vi "Create from Info.vi"(8 "error in (no error)":errorcluster, 9 "Folder":path, 10 "Package Info":T1, 11 "NamedPackage in":refnum<class "NamedPackage.lvclass">) -> (0 "error out":errorcluster, 3 "NamedPackage out":refnum<class "NamedPackage.lvclass">)   [LabVIEW 2020, in "GPack.lvlib" / "NamedPackage.lvclass"]
uses:
  NamedPackage.lvclass
  Package Info.ctl
  NamedPackage.lvclass/NamedPackage.ctl
  GPack.lvlib
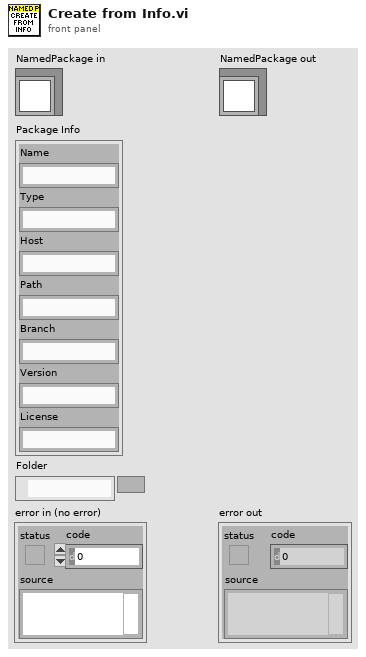
[diagram p1: front panel]
types:
  T1 = typedef "GPack.lvlib/Package Info.ctl" = cluster{"Name":string, "Type":string, "Host":string, "Path":string, "Branch":string, "Version":string, "License":string}
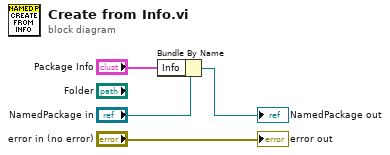
[diagram p0: block diagram]
diagram:
  n1 = Bundle By Name(cluster="NamedPackage in", "Info"="Package Info") -> (→"NamedPackage out":refnum<class "NamedPackage.lvclass">)
  "error out" <- "error in (no error)"
